vi "Check Split.vi"(8 "error in (no error)":errorcluster, 11 "Historian Logger in":refnum<class "Historian Logger.lvclass">) -> (0 "error out":errorcluster, 3 "Historian Logger out":refnum<class "Historian Logger.lvclass">)   [LabVIEW 2020, in "VolatusHistorian.lvlib" / "Historian Logger.lvclass"]
uses:
  Historian Logger.lvclass
  Historian Logger.lvclass/Historian Logger.ctl
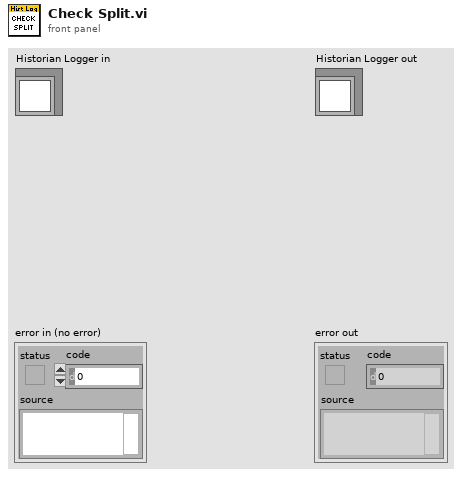
[diagram p1: front panel]
types:
  T1 = typedef "LVDateTimeRec.ctl" = cluster{"fractional second":dbl, "second":i32, "minute":i32, "hour":i32, "day of month":i32, "month":i32, "year":i32, "day of week":i32, "day of year":i32, "DST":i32}
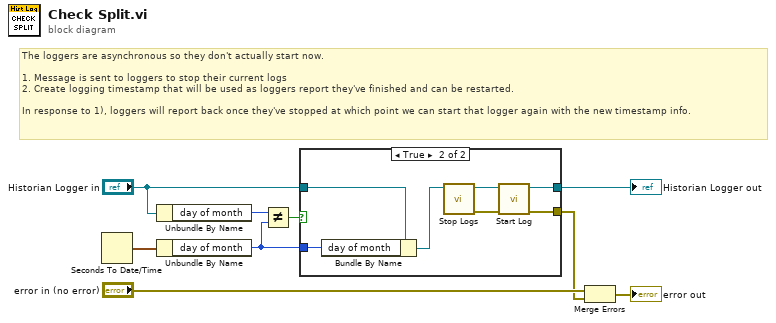
[diagram p0: block diagram]
diagram:
  # "The loggers are asynchronous so they don't actually start now.\n\n1. Message is sent to loggers to stop their current logs\n2. Create logging timestamp that will be used as loggers report they've finished and can be restarted.\n\nIn response to 1), loggers will report back once they've stopped at which point we can start that logger again with the new timestamp info."
  n1 = Seconds To Date/Time() -> (date time rec=w8:T1)  [unwired: 2 in]
  n2 = Unbundle By Name("Historian Logger in") -> ("day of month"=w7:i32)
  n3 = Unbundle By Name(w8) -> ("day of month"=w3:i32)
  n4 = Not Equal?(x=w7, y=w3) -> (x != y?=w4:bool)
  n5 = case shown="True" w4 {
    tunnel: "Historian Logger in" -> [w10 w17]
    tunnel: [w10 w12] -> w5
    tunnel: w3 -> [_ w16]
    tunnel: [_ w11] -> w1
    frame False {
    }
    frame True {
      n6 = Bundle By Name(cluster=w17, "day of month"=w16) -> (w15:refnum<class "Historian Logger.lvclass">)
      n7 = call "Stop Logs.vi"("Historian Logger in"=w15) -> ("error out"=w13:errorcluster, "Historian Logger out"=w14:refnum<class "Historian Logger.lvclass">)  [unwired: 9 in]
      n8 = call "Start Log.vi"("error in (no error)"=w13, "Historian Logger in"=w14) -> ("error out"=w11:errorcluster, "Historian Logger out"=w12:refnum<class "Historian Logger.lvclass">)  [unwired: 8 in]
    }
  }
  "Historian Logger out" <- w5
  n9 = Merge Errors("error in (no error)", w1) -> (→"error out":errorcluster)
